vi "CreateQueque.vi"(11 "queueName":string="print") -> (3 "queue":string)   [LabVIEW 2011]
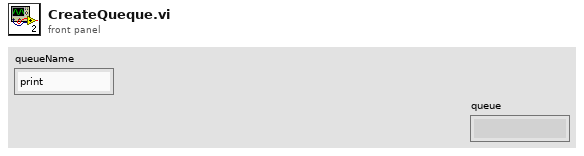
[diagram p1: front panel]
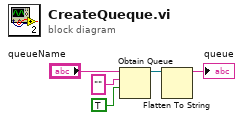
[diagram p0: block diagram]
diagram:
  n1 = Obtain Queue(name (unnamed)="queueName", element data type="" ("queueName 2"), create if not found? (T)=TRUE ("如未找到是否创建？(T)")) -> (queue out=w2:refnum<queue>)  [unwired: 2 in, 2 out]
  n2 = Flatten To String(anything=w2) -> (data string=→"queue":string)  [unwired: 3 in, 2 out]
